vi "Configure IR High Limit.vi"(7 "Mode":u16(ring) items=["IR"], 8 "error in (no error)":errorcluster, 9 "Hi Limit [ohm]":dbl min=0.0 max=50000000000.0 step=0.1 format="%.3p", 10 "Step":T1=1 min=1 max=99 step=1, 11 "VISA resource name":refnum<visa-resource-name>) -> (0 "error out":errorcluster, 3 "VISA resource name out":refnum<visa-resource-name>)   [LabVIEW 2025, in "Chroma 19052.lvlib"]
uses:
  <instrlib>/Chroma 19052/Chroma 19052.lvlib
  <instrlib>/Chroma 19052/Public/Utility/Type Def/steps--numeric.ctl
panel:
  # "Configure IR High Limit"
  # "0.1 Mohm to 10 Gohm (19053, 19054)\n0.1 Mohm to 50 Gohm (19052 only)"
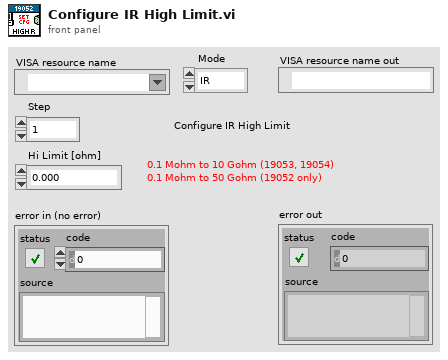
[diagram p1: front panel]
types:
  T1 = typedef "Chroma 19052.lvlib/steps--numeric.ctl" = u8
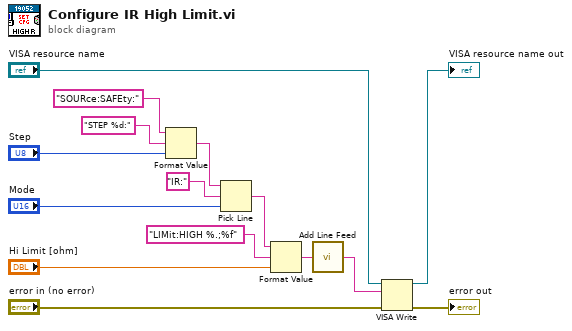
[diagram p0: block diagram]
diagram:
  n1 = Format Value(string ("")="SOURce:SAFEty:", format string="STEP %d:", value (0)="Step") -> (output string=w10:string)
  n2 = Pick Line(string ("")=w10, multi-line string="IR:", line index="Mode") -> (output string=w7:string)
  n3 = Format Value(string ("")=w7, format string="LIMit:HIGH %.;%f", value (0)="Hi Limit [ohm]") -> (output string=w6:string)
  n4 = call <instrlib>:"Add Line Feed.vi"("Command string"=w6) -> ("Concatenated string"=w5:string)  [unwired: 4 in]
  n5 = VISA Write(VISA resource name="VISA resource name", write buffer=w5, error in (no error)="error in (no error)") -> (VISA resource name out=→"VISA resource name out":refnum<visa-resource-name>, error out=→"error out":errorcluster)  [unwired: 1 out]
